vi "GenesysPS.ProcPeriodic.vi"(0 "i ref in":refnum<vi>, 3 "ms timeout (10000)":i32=10000, 5 "error in (no error)":errorcluster) -> (14 "i ref out":refnum<vi>, 17 "timed out":bool, 19 "error out":errorcluster)   [LabVIEW 2014, in "GenesysPS.lvlib"]
doc: "This method serves to periodically do things like reading values from the HW. Methods that should be executed periodically should be called from THIS methode. Add code here."
uses:
  GenesysPS.lvlib
  CSlibraries-extern/DimLVEvent/LVDimInterface/LVDimInterface.lvlib
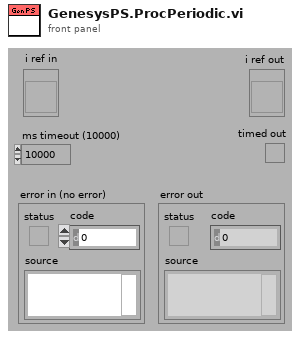
[diagram p1: front panel]
types:
  T1 = typedef "GenesysPS.lvlib/GenesysPS.i attribute.ctl" = cluster{"VISA name/ Heizinger":refnum<visa-resource-name>, "GEN Addr":i32, "WithTempInt?":bool, "TempLimit":dbl, "TemperatureID":i32, "Temp queue":refnum<queue>}
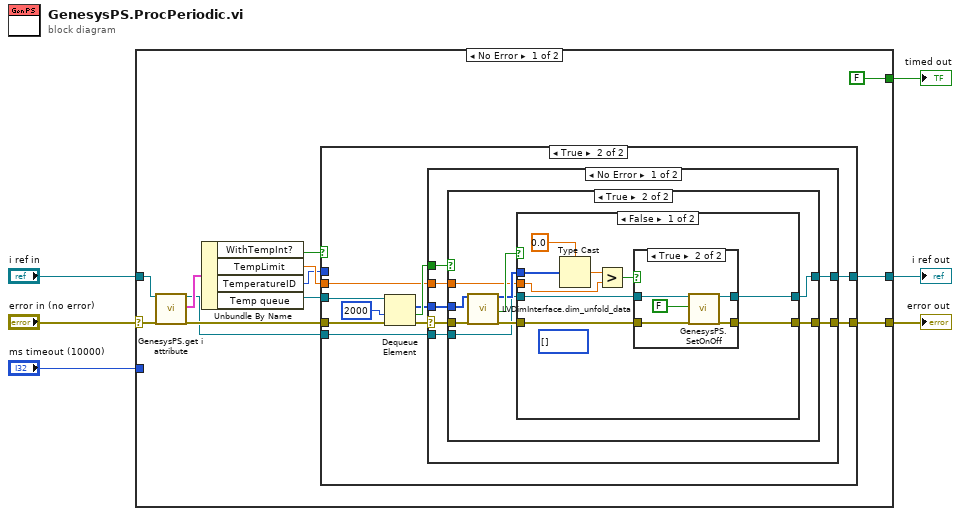
[diagram p0: block diagram]
diagram:
  n1 = case shown="No Error" "error in (no error)" {
    selector: "error in (no error)" -> [w17 w69]
    tunnel: [w12 w69] -> w5
    tunnel: "i ref in" -> [w16 w70]
    tunnel: [w7 w70] -> w3
    tunnel: [FALSE _] -> w2
    tunnel: "ms timeout (10000)" -> [_ _]
    frame No Error {
      n2 = call "GenesysPS.get i attribute.vi"("i ref in"=w16, "error in (no error)"=w17) -> ("i ref out"=w8:refnum<vi>, "i attribute"=w15:T1, "error out"=w13:errorcluster)  [unwired: 15 in]
      n3 = Unbundle By Name(w15) -> ("WithTempInt?"=w14:bool, "TempLimit"=w10:dbl, "TemperatureID"=w9:i32, "Temp queue"=w11:refnum<queue>)
      n4 = case shown="True" w14 {
        tunnel: w13 -> [w20 w29]
        tunnel: [w20 w28] -> w12
        tunnel: w11 -> [_ w27]
        tunnel: w10 -> [_ w23]
        tunnel: w9 -> [_ _]
        tunnel: w8 -> [w19 w22]
        tunnel: [w19 w21] -> w7
        frame False {
        }
        frame True {
          n5 = Dequeue Element(queue=w27, timeout in ms (-1)=2000, error in (no error)=w29) -> (element=w24:i8[], timed out?=w26:bool, error out=w25:errorcluster)  [unwired: 1 out]
          n6 = case shown="No Error" w25 {
            selector: w25 -> [w35 w68]
            tunnel: [w37 w68] -> w28
            tunnel: w26 -> [w36 _]
            tunnel: w24 -> [w34 _]
            tunnel: w23 -> [w33 _]
            tunnel: w22 -> [w32 w67]
            tunnel: [w31 w67] -> w21
            frame No Error {
              n7 = case shown="True" w36 {
                tunnel: w35 -> [w39 w48]
                tunnel: [w39 w42] -> w37
                tunnel: w34 -> [_ w47]
                tunnel: w33 -> [_ w44]
                tunnel: w32 -> [w38 w41]
                tunnel: [w38 w40] -> w31
                frame False {
                }
                frame True {
                  n8 = call "LVDimInterface.dim_unfold_data.vi"("rawData"=w47, "error in (no error)"=w48) -> ("data"=w45:i8[], "no link"=w46:bool, "error out"=w43:errorcluster)  [unwired: 14 in, 1 out]
                  n9 = case shown="False" w46 {
                    tunnel: w45 -> [w57 _]
                    tunnel: w44 -> [w54 _]
                    tunnel: w43 -> [w52 w66]
                    tunnel: [w51 w66] -> w42
                    tunnel: w41 -> [w50 w65]
                    tunnel: [w49 w65] -> w40
                    frame False {
                      (unwired) i16[] []
                      n10 = Type Cast(type=0.0, x=w57) -> (*(type *) &x=w55:dbl)
                      n11 = Greater?(x=w55, y=w54) -> (0:w53:bool)
                      n12 = case shown="True" w53 {
                        tunnel: w52 -> [w59 w64]
                        tunnel: [w59 w63] -> w51
                        tunnel: w50 -> [w58 w61]
                        tunnel: [w58 w60] -> w49
                        frame False {
                        }
                        frame True {
                          n13 = call "GenesysPS.SetOnOff.vi"("i ref in"=w61, "on (FALSE)"=FALSE, "error in (no error)"=w64) -> ("i ref out"=w60:refnum<vi>, "error out"=w63:errorcluster)  [unwired: 15 in]
                        }
                      }
                    }
                    frame True {
                    }
                  }
                }
              }
            }
            frame Error {
            }
          }
        }
      }
    }
    frame Error {
    }
  }
  "error out" <- w5
  "i ref out" <- w3
  "timed out" <- w2
